vi "Read Get Meta Data.vi"(8 "error in":errorcluster, 11 "UDP in":refnum<class "UDP.lvclass">) -> (0 "error out":errorcluster, 2 "Get Meta Data":T1, 3 "UDP out":refnum<class "UDP.lvclass">)   [LabVIEW 2020, in "Plugin Instrument Driver.lvlib" / "UDP.lvclass"]
doc: "Read get meta data"
uses:
  UDP.lvclass
  builds/Libraries/Shared GUI Library.lvlibp/Shared GUI Library/Device Meta Data Cluster/Get Meta Data.ctl
  UDP.lvclass/UDP.ctl
  builds/Libraries/Shared GUI Library.lvlibp
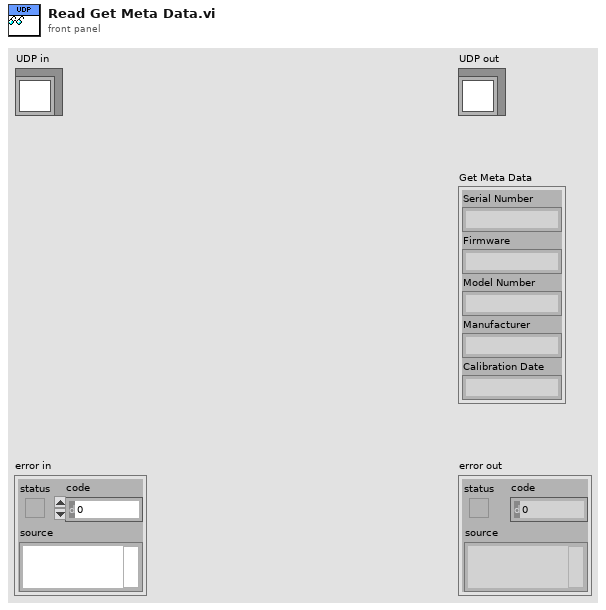
[diagram p1: front panel]
types:
  T1 = typedef "Shared GUI Library.lvlibp/Get Meta Data.ctl" = cluster{"Serial Number":string, "Firmware":string, "Model Number":string, "Manufacturer":string, "Calibration Date":string}
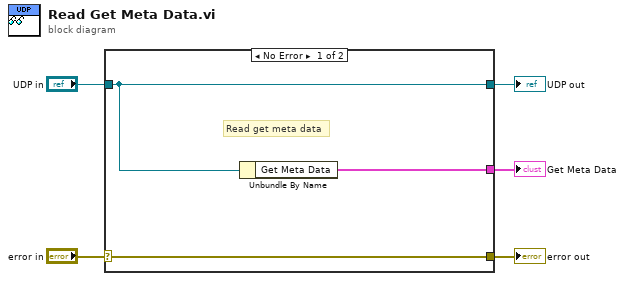
[diagram p0: block diagram]
diagram:
  n1 = case shown="No Error" "error in" {
    selector: "error in" -> [w8 w9]
    tunnel: [w8 w9] -> w4
    tunnel: [w7 w10] -> w2
    tunnel: "UDP in" -> [w7 w10]
    tunnel: [w6 _] -> w1
    frame No Error {
      # "Read get meta data"
      n2 = Unbundle By Name(w7) -> ("Get Meta Data"=w6:T1)
    }
    frame Error {
    }
  }
  "error out" <- w4
  "UDP out" <- w2
  "Get Meta Data" <- w1
